vi "run_as_admin.vi"(8 "error in (no error)":errorcluster, 10 "arguments":string, 11 "command":path) -> (0 "error out":errorcluster)   [LabVIEW 2015, in "lv-bin-windows.lvlib" / "v1.lvlib"]
uses:
  v1.lvlib
  <userlib>/antonio-alexander/lv-bin/lv-bin/public/api/v1/v1.lvlib
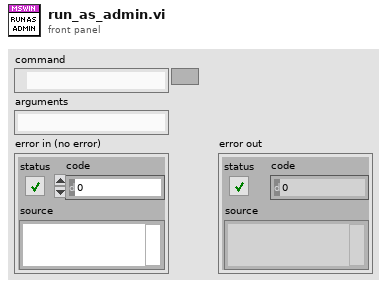
[diagram p1: front panel]
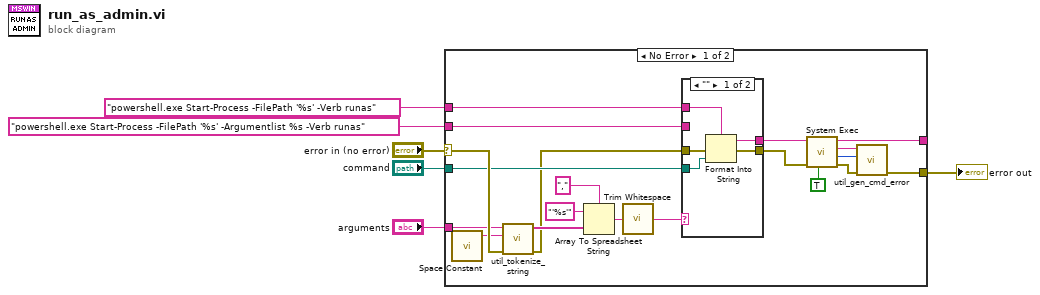
[diagram p0: block diagram]
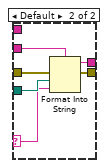
[diagram p2: hidden frame]
diagram:
  n1 = case shown="No Error" "error in (no error)" {
    selector: "error in (no error)" -> [w21 w38]
    tunnel: "powershell.exe Start-Process -FilePath '%s' -Argumentlist %s -Verb runas" ("format string") -> [w20 _]
    tunnel: [w26 w38] -> w5
    tunnel: [w25 _] -> _
    tunnel: "command" -> [w15 _]
    tunnel: "arguments" -> [w19 _]
    tunnel: "powershell.exe Start-Process -FilePath '%s' -Verb runas" ("format string") -> [w7 _]
    frame No Error {
      n2 = call <vilib>:"Space Constant.vi"() -> ("String"=w12:string)
      n3 = call <userlib>:"util_tokenize_string.vi"("error in (no error)"=w21, "delimiter"=w12, "input_string"=w19) -> ("error out"=w14:errorcluster, "before_match []"=w18:string[])  [unwired: 6 in, 1 out]
      n4 = Array To Spreadsheet String(delimiter (Tab)=",", array=w18, 3:"'%s'" ("format string")) -> (spreadsheet string=w11:string)
      n5 = call <vilib>:"Trim Whitespace.vi"("string"=w11) -> ("trimmed string"=w8:string)  [unwired: 1 in]
      n6 = case shown="\"\"" w8 {
        selector: w8 -> [_ w32]
        tunnel: [w27 w37] -> w24
        tunnel: w20 -> [_ w36]
        tunnel: w15 -> [w29 w35]
        tunnel: w14 -> [w31 w34]
        tunnel: [w30 w33] -> w13
        tunnel: w7 -> [w28 _]
        frame "" {
          n7 = Format Into String(format string=w28, error in=w31, w29) -> (resulting string=w27:string, error out=w30:errorcluster)  [unwired: 1 in]
        }
        frame Default {
          n8 = Format Into String(format string=w36, error in=w34, w35, w32) -> (resulting string=w37:string, error out=w33:errorcluster)  [unwired: 1 in]
        }
      }
      n9 = call <vilib>:"System Exec.vi"("run minimized? (F)"=TRUE, "error in (no error)"=w13, "command line"=w24) -> ("error out"=w22:errorcluster, "return code"=w9:i32, "standard error"=w10:string, "standard output"=w25:string)  [unwired: 5 in]
      n10 = call <userlib>:"util_gen_cmd_error.vi"("error in (no error)"=w22, "return_code"=w9, "standard_error"=w10) -> ("error out"=w26:errorcluster)  [unwired: 8 in]
    }
    frame Error {
    }
  }
  "error out" <- w5
